vi "Plot.vi"(0 "MRN in":refnum<class "Moving Ripple Noise.lvclass">, 11 "error in (no error)":errorcluster) -> (4 "MRN out":refnum<class "Moving Ripple Noise.lvclass">, 15 "error out":errorcluster)   [LabVIEW 2015, in "Moving Ripple Noise.lvclass"]
uses:
  Moving Ripple Noise.lvclass
  Moving Ripple Noise.lvclass/Moving Ripple Noise.ctl
  Utility VIs/Math VIs/LinSpace (start-stop-step).vi
panel:
  in  "Npts":i32
  in  "Fs (Hz)":dbl
  in  "Freq axis":dbl(slide) caption="Frequency" scale=0.0..72.0
  out "Graph":dbl[][](graph)
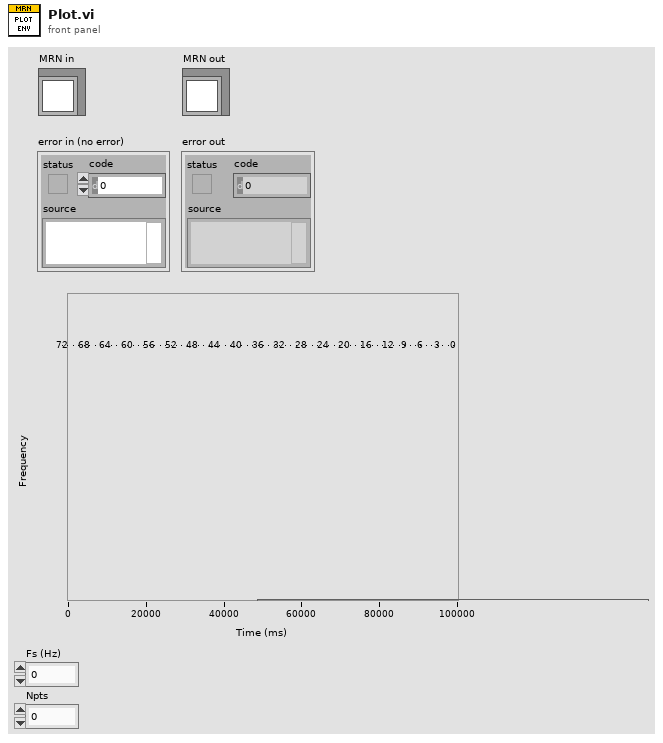
[diagram p1: front panel]
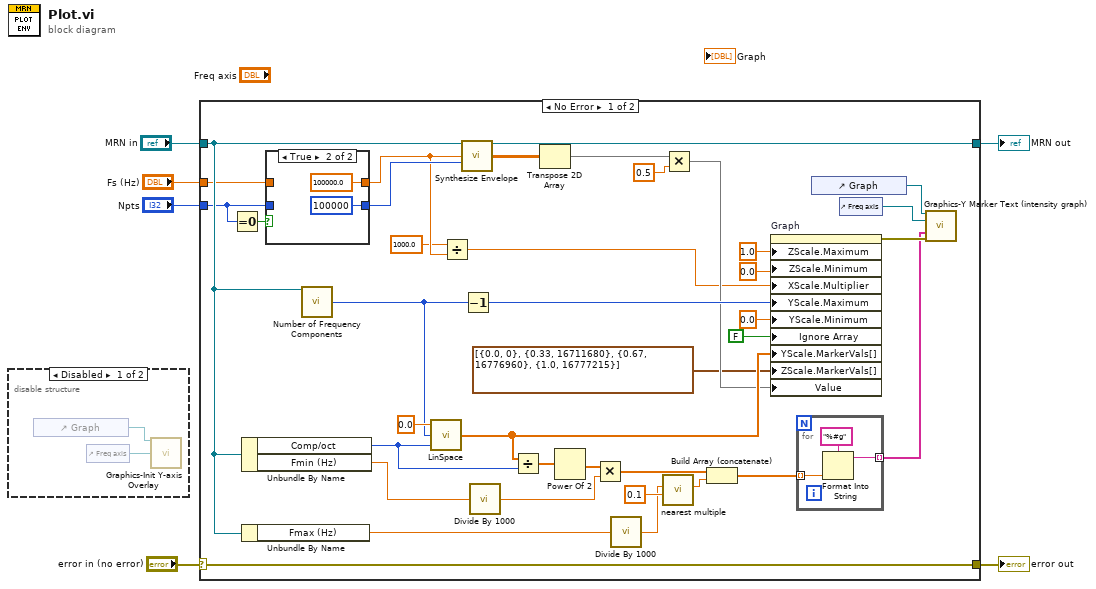
[diagram p0: block diagram]
diagram:
  n1 = disable-structure shown="Disabled" {
    frame Disabled {
      n2 = control-ref of="Graph"() -> (w8:refnum<vi>)
      n3 = control-ref of="Freq axis"() -> (w7:refnum<vi>)
      n4 = call "Graphics-Init Y-axis Overlay.vi"("Ctl Refnum"=w8, "Y-axis slider"=w7) -> ()  [unwired: 13 in, 1 out]
    }
    frame Enabled {
    }
  }
  n5 = case shown="No Error" "error in (no error)" {
    selector: "error in (no error)" -> [w46 w55]
    tunnel: [w46 w55] -> w3
    tunnel: [w29 w54] -> w5
    tunnel: "MRN in" -> [w28 w54]
    tunnel: "Fs (Hz)" -> [w15 _]
    tunnel: "Npts" -> [w13 _]
    frame No Error {
      n6 = Equal To 0?(x=w13) -> (x = 0?=w12:bool)
      n7 = Unbundle By Name(w28) -> ("Comp/oct"=w44:i32, "Fmin (Hz)"=w41:dbl)
      n8 = Unbundle By Name(w28) -> ("Fmax (Hz)"=w26:dbl)
      n9 = case shown="True" w12 {
        tunnel: w15 -> [w48 _]
        tunnel: [w48 100000.0 ("Fs (Hz)")] -> w11
        tunnel: [w47 100000 ("Npts")] -> w14
        tunnel: w13 -> [w47 _]
        frame False {
        }
        frame True {
        }
      }
      n10 = call "Number of Frequency Components.vi"("MRN in"=w28) -> ("Nfreq"=w27:i32)  [unwired: 12 in, 2 out]
      n11 = call-poly "LinSpace.vi"("Step"=w44, "Stop"=w27, "Start"=0.0 ("Y Scale.Range:Minimum")) -> ("Array"=w21:dbl[])  [unwired: 1 in, 1 out]
      n12 = Divide(x=1000.0, y=w11) -> (x/y=w9:dbl)
      n13 = call "Synthesize Envelope.vi"("MRN in"=w28, "Fs (Hz)"=w11, "Npts"=w14) -> ("MRN out"=w29:refnum<class "Moving Ripple Noise.lvclass">, "Envelope"=w25:dbl[][])  [unwired: 10 in, 1 out]
      n14 = Decrement(x=w27) -> (x-1=w22:i32)
      n15 = call "Divide By 1000.vi"("X"=w41) -> ("X/1000"=w40:dbl)
      n16 = Divide(x=w21, y=w44) -> (x/y=w43:dbl[])
      n17 = Transpose 2D Array(2D array=w25) -> (transposed array=w20:dbl[][])
      n18 = Power Of 2(x=w43) -> (2^x=w42:dbl[])
      n19 = Multiply(x=w42, y=w40) -> (x*y=w24:dbl[])
      n20 = call "Divide By 1000.vi"("X"=w26) -> ("X/1000"=w32:dbl)
      n21 = call "nearest multiple.vi"("y"=0.1, "x"=w32) -> ("round(x/y)*y"=w34:dbl)  [unwired: 7 in, 2 out]
      n22 = Multiply(x=w20, y=0.5) -> (x*y=w18:dbl[][])
      n23 = Build Array (concatenate)(w24, w34) -> (w23:dbl[])
      n24 = property on="Graph" class="IntGraph (strict)"("ZScale.Maximum"=1.0 ("Z Scale.Range:Maximum"), "ZScale.Minimum"=0.0 ("Z Scale.Range:Minimum"), "XScale.Multiplier"=w9, "YScale.Maximum"=w22, "YScale.Minimum"=0.0 ("Y Scale.Range:Minimum"), "Ignore Array"=FALSE, "YScale.MarkerVals[]"=w21, "ZScale.MarkerVals[]"=cluster{dbl, u32}[] [{0.0, 0}, {0.33, 16711680}, {0.67, 16776960}, {1.0, 16777215}] ("Z Scale.Marker Values[]"), "Value"=w18) -> (error out=w39:errorcluster)  [unwired: 2 in, 1 out]
      n25 = for {
        tunnel: w23 -> [w53] mode=indexing
        tunnel: [w52] -> w35 mode=indexing
        n26 = Format Into String(format string="%#g" ("initial string"), w53) -> (resulting string=w52:string)  [unwired: 2 in, 1 out]
      }
      n27 = control-ref of="Graph"() -> (w37:refnum<vi>)
      n28 = control-ref of="Freq axis"() -> (w36:refnum<vi>)
      n29 = call "Graphics-Y Marker Text (intensity graph).vi"("Graph"=w37, "Slider"=w36, "Text Labels[]"=w35, "error in (no error)"=w39) -> ()  [unwired: 11 in, 1 out]
    }
    frame Error {
    }
  }
  "error out" <- w3
  "MRN out" <- w5
